vi "ConfigTreeOperation(multi).vi"(8 "error in (no error)":errorcluster, 10 "Tree Refnum":refnum<vi>, 11 "configtable":T3 {"CHS"."display" format="%b"}) -> (0 "error out":errorcluster, 2 "Tree Refnum out":refnum<vi>)   [LabVIEW 2011]
uses:
  contable.ctl
  CHS.ctl
  singlechtype.ctl
  chtype.ctl
  config table enum.ctl
panel:
  in  "Tree":string(tree)
  in  "chtree config":T1={"ch"=[{"String"="通道名", "use"=TRUE, "display"=0, "Enum"=enum."Chname"}, {"String"="使用", "use"=TRUE, "display"=0, "Enum"=enum."USE"}, {"String"="频率", "use"=TRUE, "display"=0, "Enum"=enum."fre"}, {"String"="增益", "use"=TRUE, "display"=0, "Enum"=enum."range"}, {"String"="传感器型号", "use"=TRUE, "display"=0, "Enum"=enum."senNO"}, {"String"="物理量", "use"=TRUE, "display"=0, "Enum"=enum."PHname"}, {"String"="单位", "use"=TRUE, "display"=0, "Enum"=enum."unit"}, {"String"="校准类别", "use"=TRUE, "display"=0, "Enum"=enum."CALclass"}, {"String"="校准系数", "use"=TRUE, "display"=0, "Enum"=enum."K"}, {"String"="样准偏移量", "use"=TRUE, "display"=0, "Enum"=enum."OFF"}, {"String"="报警", "use"=TRUE, "display"=0, "Enum"=enum."Alrm"}, {"String"="滤波", "use"=TRUE, "display"=0, "Enum"=enum."filt"}, {"String"="电源供电", "use"=TRUE, "display"=0, "Enum"=enum."Power"}, {"String"="显示", "use"=TRUE, "display"=0, "Enum"=enum."display"}, {"String"="报警判断", "use"=TRUE, "display"=0, "Enum"=enum."compare"}, {"String"="判断值", "use"=TRUE, "display"=0, "Enum"=enum."threshold"}, {"String"="信号类型", "use"=TRUE, "display"=0, "Enum"=enum."Etype"}], "displya num"=1, "range value"=["0~10V", "0~5V", "±10V", "±5V", "", "", "", "", "", "", "", "", "", "", "", "", "", "", "", ""], "Etype"=["0~10V", "0~5V", "±10V", "±5V", "", "", "", "", "", "", "", "", "", "", "", "", "", "", "", ""], "CLASS"=[enum."CNO", enum."CName", enum."ClassI"]}
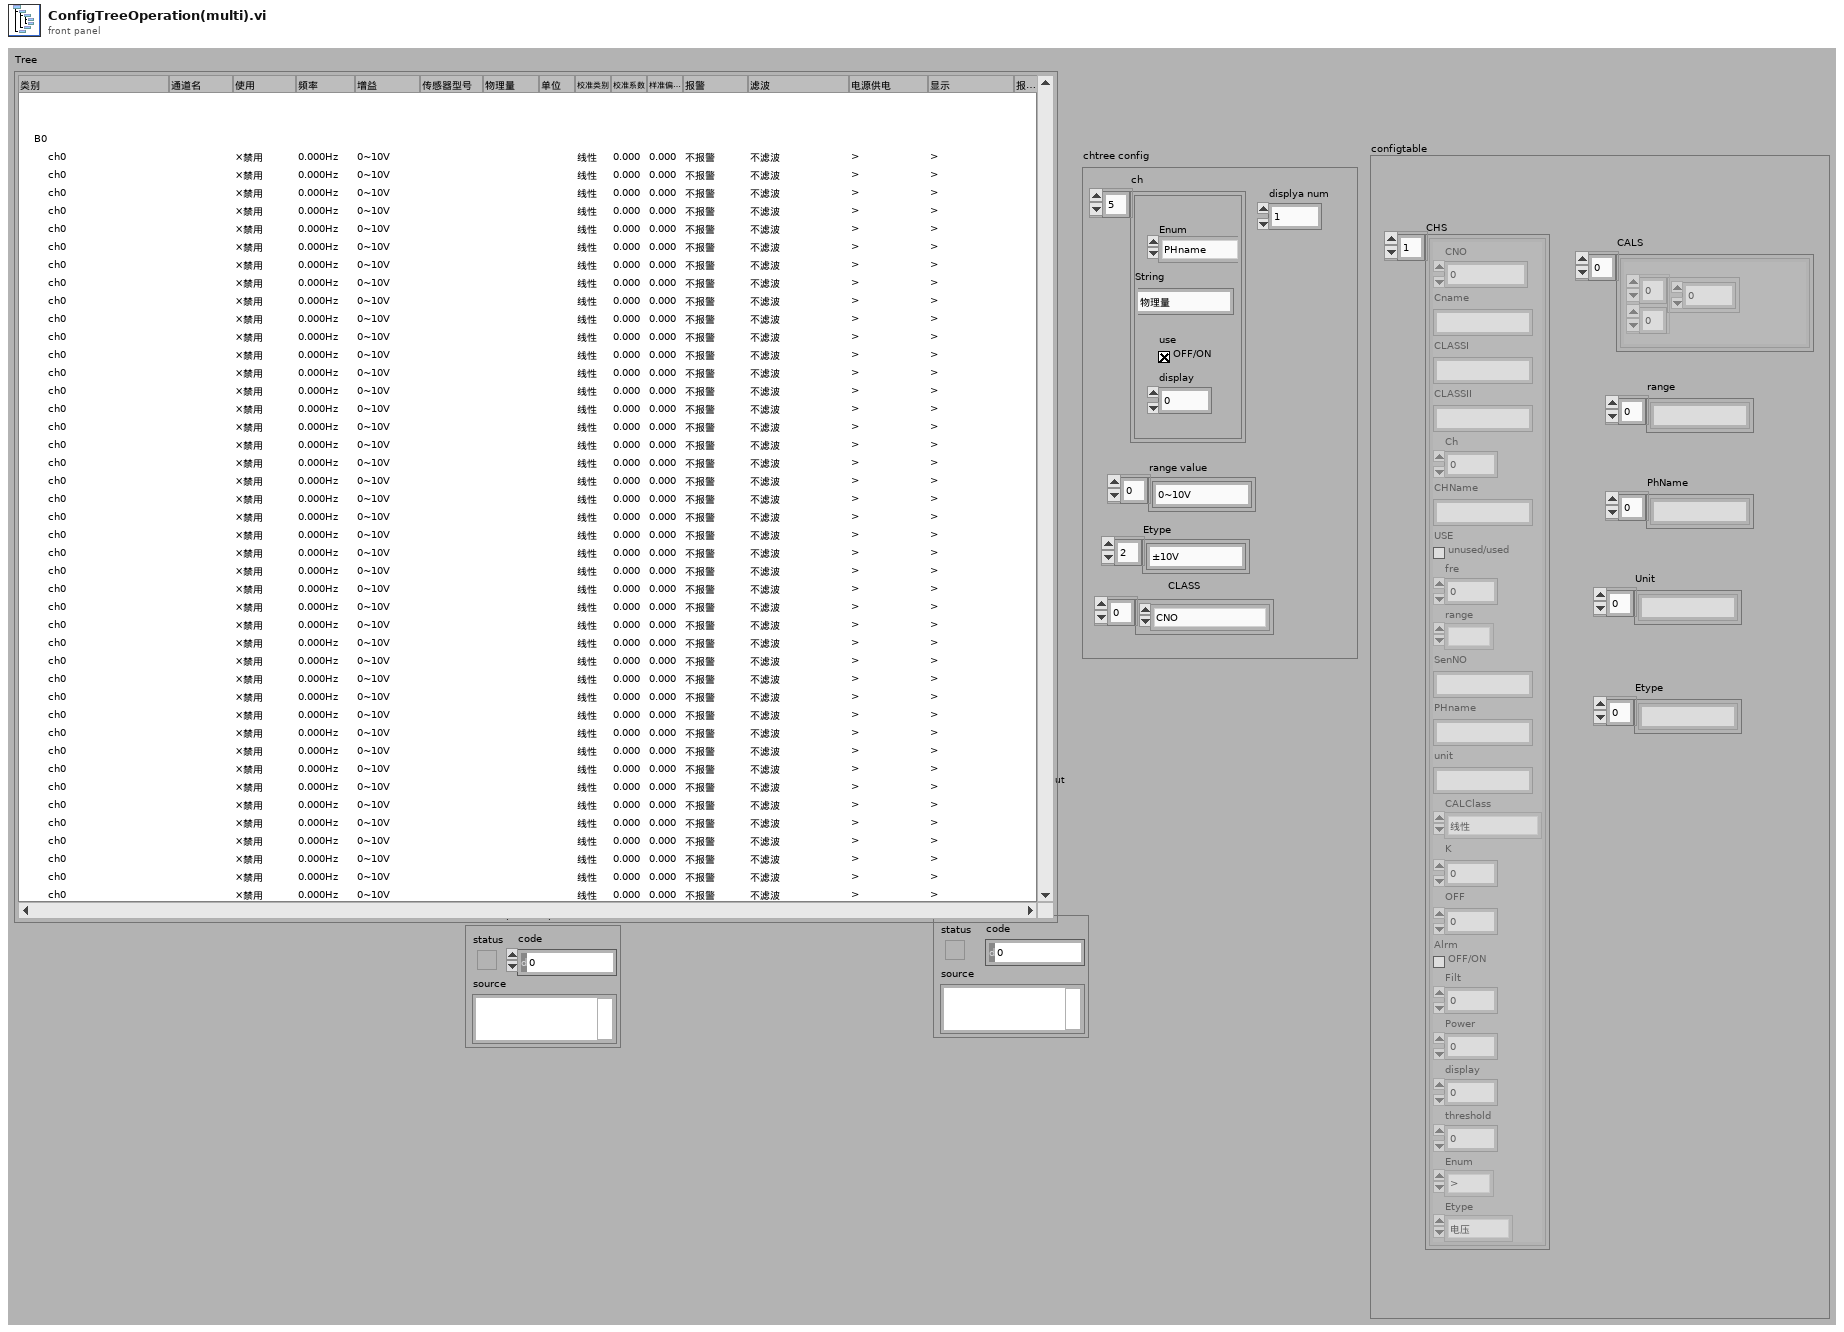
[diagram p1: front panel]
types:
  T1 = typedef "chtype.ctl" = cluster{"ch":cluster{"String":string, "use":bool, "display":u16, "Enum":T2}[], "displya num":i32, "range value":string[], "Etype":string[], "CLASS":enum16{"CName", "CNO", "ClassI", "ClassII"}[]}
  T2 = typedef "config table enum.ctl" = enum16{"CNO.", "CName", "CLASSI", "CLASSII", "ch", "Chname", "USE", "fre", "range", "senNO", "PHname", "unit", "CALclass", "K", "OFF", "Alrm", "filt", "Power", "display", "threshold", "compare", "Etype"}
  T3 = typedef "contable.ctl" = cluster{"CHS":T4, "CALS":cluster{"Array":dbl[][]}[], "range":string[], "PhName":string[], "Unit":string[], "Etype":string[]}
  T4 = typedef "CHS.ctl" = T5[]
  T5 = typedef "singlechtype.ctl" = cluster{"CNO":u8, "Cname":string, "CLASSI":string, "CLASSII":string, "Ch":u8, "CHName":string, "USE":bool, "fre":dbl, "range":enum16{""}, "SenNO":string, "PHname":string, "unit":string, "CALClass":enum8{"线性", "查表", "公式"}, "K":dbl, "OFF":dbl, "Alrm":bool, "Filt":dbl, "Power":u8, "display":u8, "threshold ":dbl, "Enum":enum16{">", ">=", "<", "<=", "<>(在范围内）", "><（在范围外）"}, "Etype":enum16{"电压", "电流", "电阻", "热电偶K", "热电偶T"}}
  T6 = typedef "chs_sort.ctl" = cluster{"sort":string, "CHS":T4}
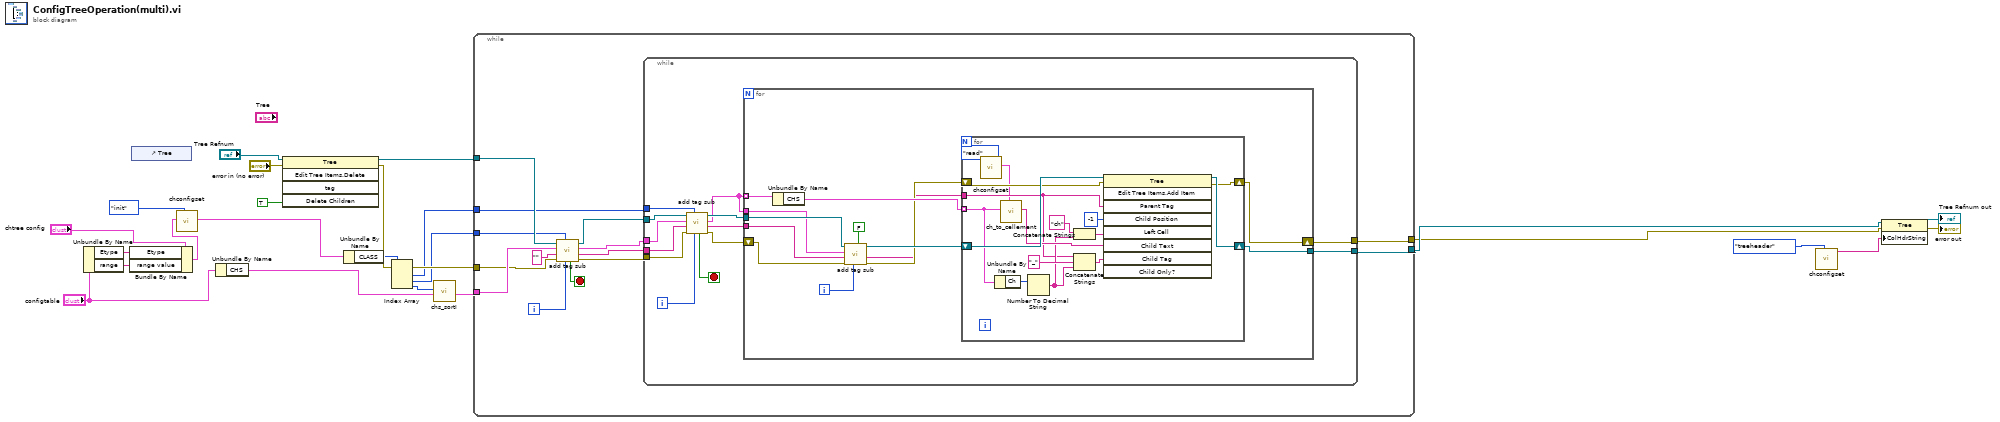
[diagram p0: block diagram]
diagram:
  n1 = Unbundle By Name("configtable") -> ("Etype"=w8:string[], "range"=w7:string[])
  n2 = Bundle By Name(cluster="chtree config", "Etype"=w8, "range value"=w7) -> (w4:T1)
  n3 = control-ref of="Tree"() -> ()  [unwired: 1 out]
  n4 = call "chconfigset.vi"("Enum"=enum16{"init", "read"}."init", "chtree config"=w4) -> ("chtree config out"=w3:T1)  [unwired: 6 in, 3 out]
  n5 = Unbundle By Name("configtable") -> ("CHS"=w17:T4)
  n6 = invoke class="Tree" method="Edit Tree Items.Delete"(reference="Tree Refnum", error in="error in (no error)", "Delete Children"=TRUE ("Delete Children?")) -> (reference out=w22:refnum<vi>, error out=w23:errorcluster)  [unwired: 2 in, 3 out]
  n7 = Unbundle By Name(w3) -> ("CLASS"=w13:enum16{"CName", "CNO", "ClassI", "ClassII"}[])
  n8 = Index Array(array=w13) -> (element #1=w19:enum16{"CName", "CNO", "ClassI", "ClassII"}, element #2=w16:enum16{"CName", "CNO", "ClassI", "ClassII"}, element #3=w18:enum16{"CName", "CNO", "ClassI", "ClassII"})  [unwired: 3 in]
  n9 = call "chs_sortI.vi"("CHS"=w17, "Enum"=w18) -> ("CH_sort"=w20:T6[])  [unwired: 9 in]
  n10 = while {
    tunnel: w23 -> [w27]
    tunnel: w22 -> [w36]
    tunnel: w20 -> [w32]
    tunnel: w19 -> [w30]
    tunnel: w16 -> [w29]
    tunnel: [w26] -> w15
    tunnel: [w25] -> w12
    i -> [w33]
    stop <- w31 stop-if-true
    n11 = call "add tag sub.vi"("index"=w33, "sort Enum"=w29, "error in (no error)"=w27, "Parent Tag"="", "CH_sort in"=w32, "reference"=w36) -> ("error out"=w38:errorcluster, "child tag"=w37:string, "CH_sort"=w28:T6[], "reference out"=w35:refnum<vi>, "stop?"=w31:bool)  [unwired: 1 in]
    n12 = while {
      tunnel: w38 -> [w47]
      tunnel: w35 -> [w50]
      tunnel: [w41] -> w26
      tunnel: [w51] -> w25
      tunnel: w28 -> [w48]
      tunnel: w37 -> [w40]
      tunnel: w30 -> [w42]
      i -> [w44]
      stop <- w43 stop-if-true
      n13 = call "add tag sub.vi"("index"=w44, "sort Enum"=w42, "error in (no error)"=w47, "Parent Tag"=w40, "CH_sort in"=w48, "reference"=w50) -> ("error out"=w46:errorcluster, "child tag"=w45:string, "CH_sort"=w39:T6[], "reference out"=w49:refnum<vi>, "stop?"=w43:bool)  [unwired: 1 in]
      n14 = for {
        tunnel: w49 -> [w60]
        tunnel: [w62] -> w41
        shift-right: [w61] -> w51
        shift-left: w46 -> [w56]
        tunnel: w39 -> [w64] mode=indexing
        tunnel: w45 -> [w57]
        tunnel: w39 -> [w58]
        i -> [w54]
        n15 = Unbundle By Name(w64) -> ("CHS"=w63:T4)
        n16 = call "add tag sub.vi"("Class"=FALSE, "index"=w54, "error in (no error)"=w56, "Parent Tag"=w57, "CH_sort in"=w58, "reference"=w60) -> ("error out"=w55:errorcluster, "child tag"=w52:string, "reference out"=w59:refnum<vi>)  [unwired: 1 in, 2 out]
        n17 = for {
          tunnel: w63 -> [w75] mode=indexing
          shift-right: [w78] -> w62
          shift-left: w59 -> [w80]
          shift-right: [w76] -> w61
          shift-left: w55 -> [w79]
          tunnel: w52 -> [w67]
          n18 = call "chconfigset.vi"("Enum"=enum16{"init", "read"}."read") -> ("chtree config out"=w66:T1)  [unwired: 7 in, 3 out]
          n19 = Unbundle By Name(w75) -> ("Ch"=w74:u8)
          n20 = call "ch_to_cellement.vi"("chtree config"=w66, "element"=w75) -> ("chtree cell Array"=w77:string[])  [unwired: 9 in]
          n21 = Number To Decimal String(number=w74) -> (decimal integer string=w70:string)  [unwired: 1 in]
          n22 = Concatenate Strings("ch" ("string"), w70) -> (w69:string)
          n23 = Concatenate Strings(w67, "_" ("string"), w70) -> (w71:string)
          n24 = invoke class="Tree" method="Edit Tree Items.Add Item"(reference=w80, error in=w79, "Parent Tag"=w67, "Child Position"=-1, "Left Cell"=w69, "Child Text"=w77, "Child Tag"=w71) -> (reference out=w78:refnum<vi>, error out=w76:errorcluster)  [unwired: 2 in, 7 out]
        }
      }
    }
  }
  n25 = call "chconfigset.vi"("Enum"=enum16{"init", "read", "treeheader"}."treeheader") -> ("tree header"=w2:string[])  [unwired: 7 in, 3 out]
  n26 = property class="Tree"(reference=w15, error in=w12, "ColHdrString"=w2) -> (reference out=→"Tree Refnum out":refnum<vi>, error out=→"error out":errorcluster)
